vi "Create Global MetaData Channel - Array - Format.vi"(8 "Error In":errorcluster, 9 "Settings":T2, 10 "Name":string, 11 "Instrument Addon Refnum In":T1=18446744073709551615 format="%.0x") -> (0 "Error Out":errorcluster, 1 "Channel Refnums":T1[](array[typedef]) format="%.0x", 2 "Array Refnum":T1 format="%.0x", 3 "Instrument Addon Refnum Out":T1=18446744073709551615 format="%.0x")   [LabVIEW 2018, in "Instrument Addon Scripting API.lvlib"]
uses:
  Instrument Addon Scripting API.lvlib
  <vilib>/NI Veristand/Custom Device API/Custom Device Item Ref.ctl
  TypeDefs/Array Format Settings.ctl
  TypeDefs/Array Element.ctl
  Addon/Addon Shared/Types/MetaData Parameters.ctl
  Addon/Addon Shared/Types/Protocol Data Type.ctl
  Addon/Addon Shared/Types/Metadata Channel Type.ctl
  Addon/Addon Shared/Types/Type Cast Type.ctl
  Addon/Addon Shared/Types/Endian.ctl
  TypeDefs/MetaData Type.ctl
  Addon/Addon Shared/Instrument Addon Shared.lvlib
  <vilib>/NI Veristand/Custom Device API/Custom Device API.lvlib
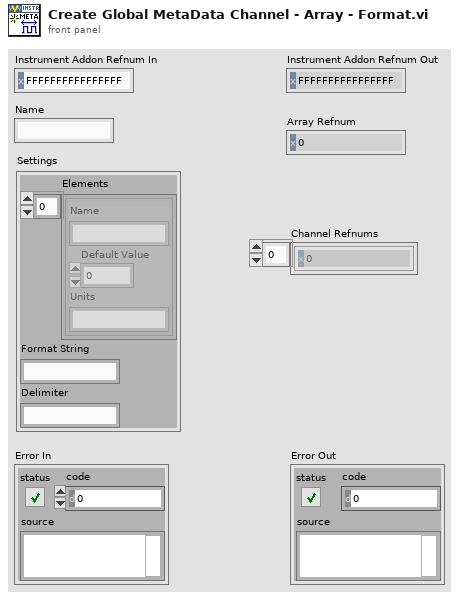
[diagram p1: front panel]
types:
  T1 = typedef "Custom Device API.lvlib/Custom Device Item Ref.ctl" = u64
  T2 = typedef "Instrument Addon Scripting API.lvlib/Array Format Settings.ctl" = cluster{"Elements":T3[], "Format String":string, "Delimiter":string}
  T3 = typedef "Instrument Addon Scripting API.lvlib/Array Element.ctl" = cluster{"Name":string, "Default Value":dbl, "Units":string}
  T4 = typedef "Instrument Addon Scripting API.lvlib/MetaData Type.ctl" = enum16{"MetaData", "Global MetaData"}
  T5 = typedef "Instrument Addon Shared.lvlib/Metadata Channel Type.ctl" = enum16{"Enumerated List", "Format", "Type Cast"}
  T6 = typedef "Instrument Addon Shared.lvlib/Protocol Data Type.ctl" = enum16{"Single Channel", "Array"}
  T7 = typedef "Instrument Addon Shared.lvlib/MetaData Parameters.ctl" = cluster{"Data Type":T6, "Channel Type":T5, "List":string[], "Format String":string, "Type":T8, "Delimiter":string, "Endian":T9}
  T8 = typedef "Instrument Addon Shared.lvlib/Type Cast Type.ctl" = enum16{"DBL", "SGL", "U64", "U32", "U16", "U8", "I64", "I32", "I16", "I8"}
  T9 = typedef "Instrument Addon Shared.lvlib/Endian.ctl" = enum16{"Native", "Little", "Big"}
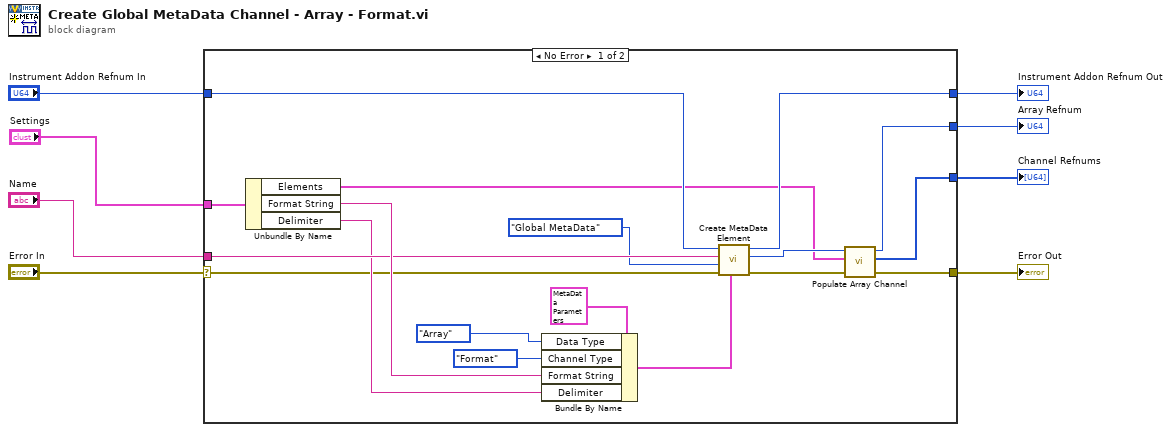
[diagram p0: block diagram]
diagram:
  n1 = case shown="No Error" "Error In" {
    selector: "Error In" -> [w14 w27]
    tunnel: "Instrument Addon Refnum In" -> [w21 w28]
    tunnel: [w20 w28] -> w7
    tunnel: "Name" -> [w19 _]
    tunnel: "Settings" -> [w18 _]
    tunnel: [w15 w27] -> w5
    tunnel: [w11 _] -> w2
    tunnel: [w10 _] -> w1
    frame No Error {
      n2 = Unbundle By Name(w18) -> ("Elements"=w12:T3[], "Format String"=w23:string, "Delimiter"=w17:string)
      n3 = Bundle By Name(cluster=T7 {"Data Type"=enum."Single Channel", "Channel Type"=enum."Format", "List"=[], "Format String"="%.3g", "Type"=enum."SGL", "Delimiter"="", "Endian"=enum."Native"} ("MetaData Parameters"), "Data Type"=Protocol_Data_Type."Array", "Channel Type"=Metadata_Channel_Type."Format", "Format String"=w23, "Delimiter"=w17) -> (w22:T7)
      n4 = call "Create MetaData Element.vi"("MetaData Parameters"=w22, "error in (no error)"=w14, "Type"=MetaData_Type."Global MetaData", "Name"=w19, "Refnum In"=w21) -> ("error out"=w16:errorcluster, "Channel Refnum"=w13:T1, "Refnum Out"=w20:T1)  [unwired: 4 in]
      n5 = call "Populate Array Channel.vi"("error in (no error)"=w16, "Elements"=w12, "Array Refnum In"=w13) -> ("error out"=w15:errorcluster, "Channel Refnums"=w11:T1[], "Array Refnum Out"=w10:T1)  [unwired: 6 in]
    }
    frame Error {
    }
  }
  "Instrument Addon Refnum Out" <- w7
  "Error Out" <- w5
  "Channel Refnums" <- w2
  "Array Refnum" <- w1
